vi "result generate filename.vi"(8 "measdata definition":T5 {"Current Magnetic\nField\n(430 TCP reading)"."phi (deg)" format="%#_3g"}, 9 "vna s-parameters":T1, 10 "sort index":i32, 11 "measurement definition":T2={"sweep parameter"=enum."angle", "sweep start"=0.0, "sweep stop"=0.0, "sweep increment"=0.0, "temperature"=0.0, "path"=path "", "magnet initial"={"magnitude"=0.0, "phi"=0.0, "theta"=0.0}, "magnet reference"={"magnitude"=0.0, "phi"=0.0, "theta"=0.0}, "const phi?"=FALSE, "delta phi (deg)"=0.5, "delta H (mT)"=0.5}) -> (3 "result path":path)   [LabVIEW 2013]
uses:
  measdata cluster.ctl
  devices/magnet/magnet polar field.ctl
  measurement sweep parameter.ctl
  devices/magnet/AMI reading polar field.ctl
  measconfig cluster.ctl
  devices/vna/vna s-parameters.ctl
panel:
  # "List of measurement data for the S-parameters."
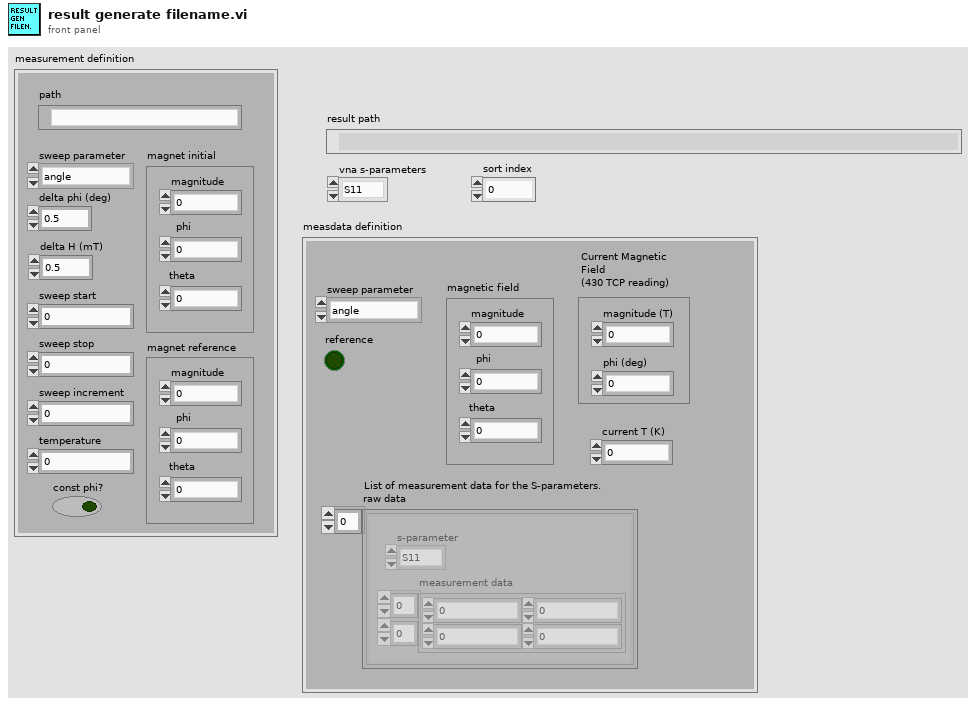
[diagram p1: front panel]
types:
  T1 = typedef "vna s-parameters.ctl" = enum16{"S11", "S12", "S21", "S22"}
  T2 = typedef "measconfig cluster.ctl" = cluster{"sweep parameter":T3, "sweep start":dbl, "sweep stop":dbl, "sweep increment":dbl, "temperature":dbl, "path":path, "magnet initial":T4, "magnet reference":T4, "const phi?":bool, "delta phi (deg)":dbl, "delta H (mT)":dbl}
  T3 = typedef "measurement sweep parameter.ctl" = enum16{"angle", "magnetic field"}
  T4 = typedef "magnet polar field.ctl" = cluster{"magnitude":dbl, "phi":dbl, "theta":dbl}
  T5 = typedef "measdata cluster.ctl" = cluster{"raw data":cluster{"measurement data":dbl[][], "s-parameter":enum16{"S11", "S12", "S21", "S22"}}[], "magnetic field":T4, "reference":bool, "sweep parameter":T3, "Current Magnetic\nField\n(430 TCP reading)":T6, "current T (K)":dbl}
  T6 = typedef "AMI reading polar field.ctl" = cluster{"magnitude (T)":dbl, "phi (deg)":dbl}
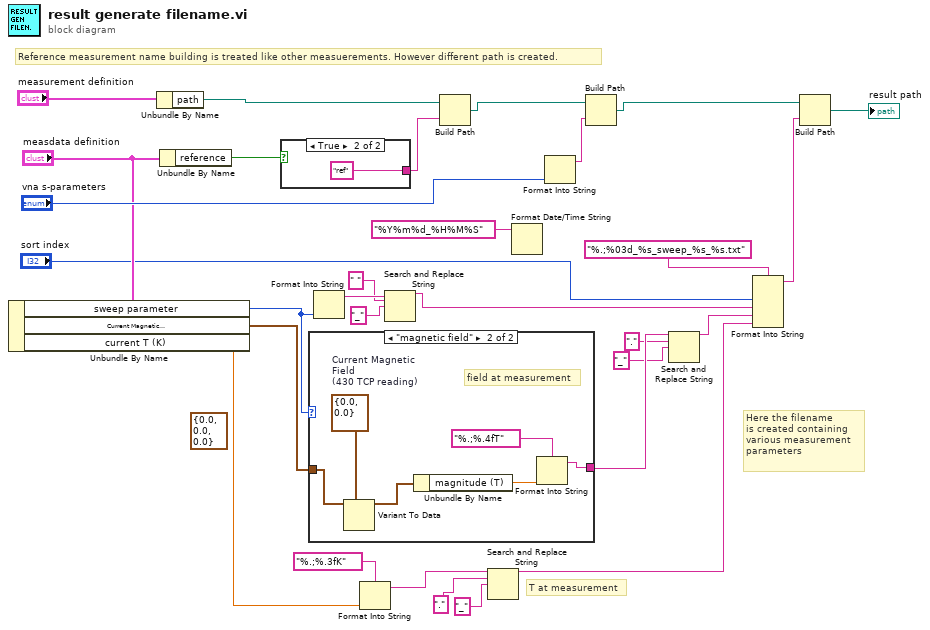
[diagram p0: block diagram]
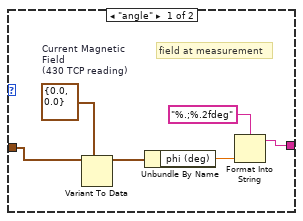
[diagram p2: hidden frame]
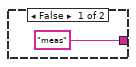
[diagram p3: hidden frame]
diagram:
  (unwired) T4 {"magnitude"=0.0, "phi"=0.0, "theta"=0.0} ("magnet polar")
  # "Here the filename \nis created containing \nvarious measurement \nparameters"
  # "Reference measurement name building is treated like other measuerements. However different path is created."
  # "T at measurement"
  n1 = Unbundle By Name("measdata definition") -> ("sweep parameter"=w18:T3, "Current Magnetic\nField\n(430 TCP reading)"=w9:T6, "current T (K)"=w7:dbl)
  n2 = Unbundle By Name("measurement definition") -> ("path"=w11:path)
  n3 = Unbundle By Name("measdata definition") -> ("reference"=w27:bool)
  n4 = case shown="True" w27 {
    tunnel: ["meas" ("name or relative path") "ref" ("name or relative path")] -> w26
    frame False {
    }
    frame True {
    }
  }
  n5 = case shown="\"magnetic field\"" w18 {
    tunnel: [w37 w42] -> w17
    tunnel: w9 -> [w35 w39]
    frame "angle" {
      w36 = T6 {"magnitude (T)"=0.0, "phi (deg)"=0.0}  # Current Magnetic Field (430 TCP reading)
      # "field at measurement"
      n6 = Variant To Data(type=w36, Variant=w35) -> (data=w34:T6)  [unwired: 1 in, 1 out]
      n7 = Unbundle By Name(w34) -> ("phi (deg)"=w33:dbl)
      n8 = Format Into String(format string="%.;%.2fdeg", w33) -> (resulting string=w37:string)  [unwired: 2 in, 1 out]
    }
    frame "magnetic field" {
      w41 = T6 {"magnitude (T)"=0.0, "phi (deg)"=0.0}  # Current Magnetic Field (430 TCP reading)
      # "field at measurement"
      n9 = Variant To Data(type=w41, Variant=w39) -> (data=w43:T6)  [unwired: 1 in, 1 out]
      n10 = Unbundle By Name(w43) -> ("magnitude (T)"=w40:dbl)
      n11 = Format Into String(format string="%.;%.4fT", w40) -> (resulting string=w42:string)  [unwired: 2 in, 1 out]
    }
  }
  n12 = Format Into String(w18) -> (resulting string=w21:string)  [unwired: 3 in, 1 out]
  n13 = Format Into String(format string="%.;%.3fK", w7) -> (resulting string=w4:string)  [unwired: 2 in, 1 out]
  n14 = Search and Replace String(input string=w21, search string=" ", replace string="_" ("replace string (\"\")")) -> (result string=w2:string)  [unwired: 5 in, 3 out]
  n15 = Build Path(base path=w11, name or relative path=w26) -> (appended path=w23:path)
  n16 = Search and Replace String(input string=w4, search string=".", replace string="_" ("replace string (\"\")")) -> (result string=w3:string)  [unwired: 5 in, 3 out]
  n17 = Format Date/Time String(time format string (%c)="%Y%m%d_%H%M%S") -> ()  [unwired: 2 in, 1 out]
  n18 = Format Into String("vna s-parameters") -> (resulting string=w24:string)  [unwired: 3 in, 1 out]
  n19 = Build Path(base path=w23, name or relative path=w24) -> (appended path=w14:path)
  n20 = Search and Replace String(input string=w17, search string=".", replace string="_" ("replace string (\"\")")) -> (result string=w10:string)  [unwired: 5 in, 3 out]
  n21 = Format Into String(format string="%.;%03d_%s_sweep_%s_%s.txt", "sort index", w2, w10, w3) -> (resulting string=w13:string)  [unwired: 2 in, 1 out]
  n22 = Build Path(base path=w14, name or relative path=w13) -> (appended path=→"result path":path)
